vi "LV SCISDK Get Components List.vi"(8 "error in (no error)":errorcluster, 9 "handle":u64, 10 "Type":string, 11 "Name":string) -> (0 "error out":errorcluster, 1 "function return":i32, 2 "ret out 2":T1(array[cluster])=[{"path"=" ", "name"="", "type"=""}])   [LabVIEW 2021, in "SciSDK_Labview.lvlib"]
doc: "SCISDKLABVIEW_DLL_API int LV_SCISDK_GetParameterString(char* Path, char* value, void* handle);"
uses:
  SciSDK_Labview.lvlib
panel:
  in  "ret in":T1(array[cluster])=[{"path"=" ", "name"="", "type"=""}]
  out "handle out":u64
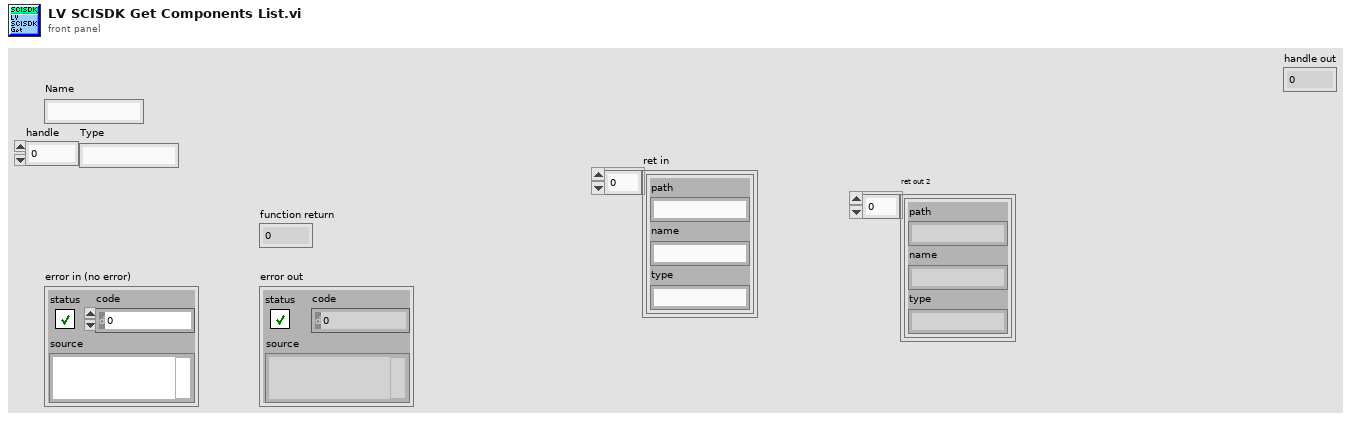
[diagram p1: front panel]
types:
  T1 = cluster{"path":string, "name":string, "type":string}[]
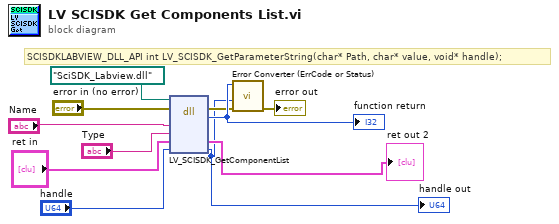
[diagram p0: block diagram]
diagram:
  # "SCISDKLABVIEW_DLL_API int LV_SCISDK_GetParameterString(char* Path, char* value, void* handle);"
  n1 = dll-call lib="C:/git/scisdk/SciSDK_VC++/x64/Debug/SciSDK_Labview.dll" fn="LV_SCISDK_GetComponentList"(path in=path "SciSDK_Labview.dll", error in="error in (no error)", "Path"="Name", "type"="Type", "ret"="ret in", "handle"="handle") -> (error out=w8:errorcluster, "return type"=w11:i32, "ret"=→"ret out 2":T1, "handle"=w1:u64)  [unwired: 3 in, 1 out]
  "function return" <- w11
  "handle out" <- w1
  n2 = call "Error Converter (ErrCode or Status).vi"("error in (no error)"=w8, "handle"=w1, "error code"=w11) -> ("error out"=→"error out":errorcluster)  [unwired: 8 in]
